vi "Create.vi"(8 "error in (no error)":errorcluster, 11 "TCP in":refnum<class "TCP.lvclass">) -> (0 "error out":errorcluster, 3 "TCP out":refnum<class "TCP.lvclass">)   [LabVIEW 2021, in "TCP.lvclass"]
uses:
  TCP.lvclass
  D:/my_projects/projects/Algorithms/Labview/21/Master CR/Master CR.lvclass
  Param/TCP Param/TCP Param.lvclass
  D:/my_projects/projects/Algorithms/Labview/21/Master CR/Param/Param.lvclass
  Master CR.lvclass/Master CR.ctl
  Master CR.lvclass
  TCP.lvclass/TCP.ctl
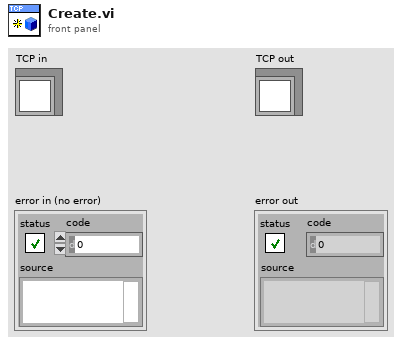
[diagram p1: front panel]
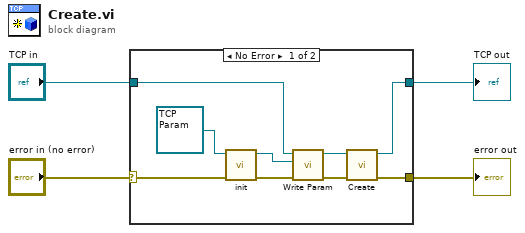
[diagram p0: block diagram]
diagram:
  n1 = case shown="No Error" "error in (no error)" {
    selector: "error in (no error)" -> [w10 w14]
    tunnel: [w5 w14] -> w1
    tunnel: [w6 w15] -> w2
    tunnel: "TCP in" -> [w9 w15]
    frame No Error {
      n2 = call-dynamic "init.vi"("error in"=w10, "Param in"=refnum<class "TCP Param.lvclass"> refnum ("Param.lvlib:TCP Param.lvclass")) -> ("error"=w11:errorcluster, "Param out"=w12:refnum<class "TCP Param.lvclass">)  [unwired: 8 in]
      n3 = call "Write Param.vi"("error in (no error)"=w11, "Param"=w12, "MB_TCP in"=w9) -> ("error out"=w7:errorcluster, "MB_TCP out"=w8:refnum<class "TCP.lvclass">)  [unwired: 7 in]
      n4 = call-parent "Create.vi"("error in (no error)"=w7, "MB in"=w8) -> ("error out"=w5:errorcluster, "MB out"=w6:refnum<class "TCP.lvclass">)  [unwired: 8 in]
    }
    frame Error {
    }
  }
  "error out" <- w1
  "TCP out" <- w2
